vi "Pre Launch Init.vi"(11 "NI_DAQmx(Angular) in":refnum<class "NI_DAQmx(Angular).lvclass">) -> (0 "error out":errorcluster, 3 "NI_DAQmx(Angular) out":refnum<class "NI_DAQmx(Angular).lvclass">)   [LabVIEW 2025, in "NI_DAQmx(Angular).lvclass"]
doc: "<p>(<strong>Filename</strong>: <span class=\"dnl\">Actor Framework.lvlib:Actor.lvclass:Pre Launch Init.vi</span>)</p>\n<p>Defines behavior that occurs after the <a href=\"nihelplauncher://docs/csh?context=lvcore_lvcomm_af_launch_nested_actor\">Launch Nested Actor</a> method is invoked but before the actor's Actor Core method begins running.</p>\n<p>By default, this method does nothing. A descendant class may override it to define behavior.</p>"
uses:
  NI_DAQmx(Angular).lvclass
  NI_DAQmx(Angular).lvclass/NI_DAQmx(Angular).ctl
  DAQ_Abstr/Task_Type/Angular_Task/Angular_Task/Angular_Task.lvclass
  <resource>/objmgr/daqmx.rc
  <vilib>/DAQmx/configure/timing.llb/DAQmx Timing (Sample Clock).vi
  <vilib>/DAQmx/create/channels.llb/DAQmx Create Channel (CI-Position-Angular Encoder).vi
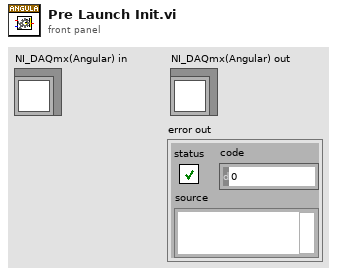
[diagram p1: front panel]
types:
  T1 = typedef "DAQ_Module.lvlib/DAQ_Module.lvclass/DAQ_Task_Config.ctl" = cluster{"Drive":T2, "TaskType":T3, "PhysicalChannels":string, "SampleRateConfiguration":T4, "ChannelConfig":string, "Enable":bool, "ShowPanel":bool}
  T2 = typedef "DAQ_Module.lvlib/DAQ_Module.lvclass/DAQ_HW_Type.ctl" = enum16{"NI_DAQmx", "Simulated_DAQ"}
  T3 = typedef "DAQ_Module.lvlib/DAQ_Module.lvclass/DAQ_Task_Type.ctl" = enum16{"AI", "Linear", "Angular", "AO"}
  T4 = typedef "DAQ_Module.lvlib/DAQ_Module.lvclass/DAQ_SampleRateConfig.ctl" = cluster{"SampleRate":dbl, "SamplesPerChannel":u32, "SamplesPerRead":i32, "SampleMode":i32, "Clock Source":string}
  T5 = typedef "DAQ_Module.lvlib/DAQ_Module.lvclass/DAQ_Angular_Task_Config.ctl" = cluster{"decoding type":i32, "units":i32, "pulses per revolution":u32, "initial angle":dbl, "z index enable":bool, "z index value":dbl, "z index phase":i32, "CI_Encoder_A_InputTerm":string, "CI_Encoder_B_InputTerm":string, "CI_Encoder_Z_InputTerm":string}
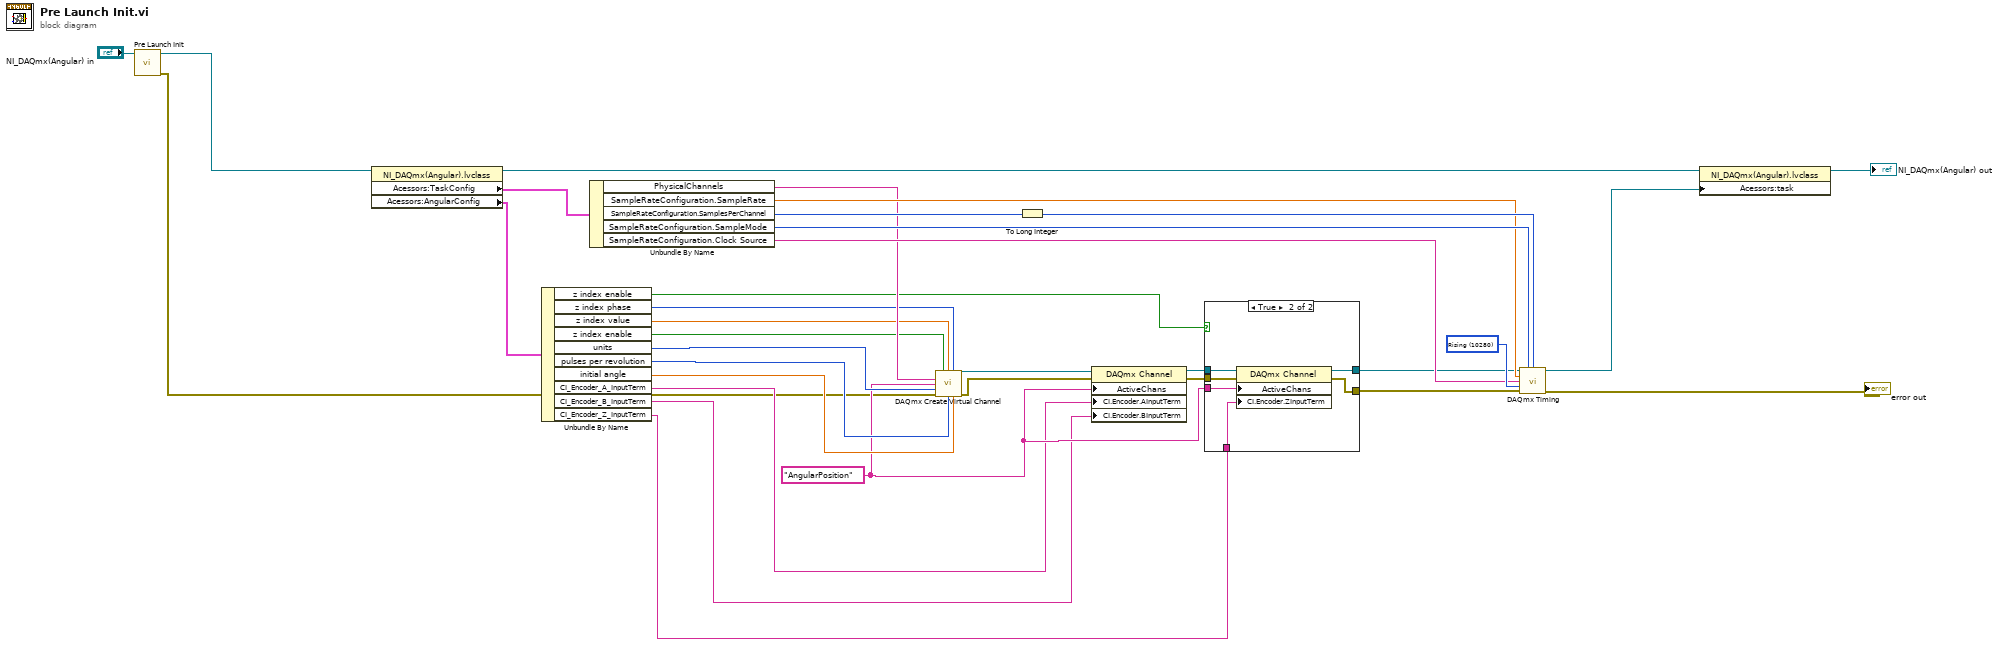
[diagram p0: block diagram]
diagram:
  w8 = "AngularPosition" ("channel name")
  w25 = 10280 items=["Rising"=10280, "Falling"=10171] ("active edge")
  n1 = call-parent "Pre Launch Init.vi"("Task_Abstr in"="NI_DAQmx(Angular) in") -> ("error out"=w1:errorcluster, "Task_Abstr out"=w4:refnum<class "NI_DAQmx(Angular).lvclass">)  [unwired: 9 in]
  n2 = property class="NI_DAQmx(Angular).lvclass"(reference=w4) -> (reference out=w32:refnum<class "NI_DAQmx(Angular).lvclass">, "Acessors:TaskConfig"=w30:T1, "Acessors:AngularConfig"=w31:T5)  [unwired: 1 in, 1 out]
  n3 = Unbundle By Name(w31) -> ("z index enable"=w9:bool, "z index phase"=w21:i32, "z index value"=w20:dbl, "z index enable"=w19:bool, "units"=w18:i32, "pulses per revolution"=w17:u32, "initial angle"=w16:dbl, "CI_Encoder_A_InputTerm"=w7:string, "CI_Encoder_B_InputTerm"=w6:string, "CI_Encoder_Z_InputTerm"=w5:string)
  n4 = Unbundle By Name(w30) -> ("PhysicalChannels"=w22:string, "SampleRateConfiguration.SampleRate"=w26:dbl, "SampleRateConfiguration.SamplesPerChannel"=w28:u32, "SampleRateConfiguration.SampleMode"=w29:i32, "SampleRateConfiguration.Clock Source"=w24:string)
  n5 = call-poly <vilib>:"DAQmx Create Virtual Channel.vi"("z index enable"=w19, "z index value"=w20, "z index phase"=w21, "counter"=w22, "name to assign"=w8, "units"=w18, "error in"=w1, "pulses per revolution"=w17, "initial angle"=w16) -> ("task out"=w13:refnum<k21>, "error out"=w11:errorcluster)  [unwired: 5 in]
  n6 = To Long Integer(number=w28) -> (32bit integer=w27:i32)
  n7 = property class="DAQmx Channel"(reference=w13, error in=w11, "ActiveChans"=w8, "CI.Encoder.AInputTerm"=w7, "CI.Encoder.BInputTerm"=w6) -> (reference out=w15:refnum<k21>, error out=w14:errorcluster)
  n8 = case shown="True" w9 {
    tunnel: w15 -> [w35 w41]
    tunnel: w14 -> [w34 w40]
    tunnel: [w34 w39] -> w10
    tunnel: [w35 w38] -> w12
    tunnel: w8 -> [_ w37]
    tunnel: w5 -> [_ w36]
    frame False {
    }
    frame True {
      n9 = property class="DAQmx Channel"(reference=w41, error in=w40, "ActiveChans"=w37, "CI.Encoder.ZInputTerm"=w36) -> (reference out=w38:refnum<k21>, error out=w39:errorcluster)
    }
  }
  n10 = call-poly <vilib>:"DAQmx Timing.vi"("task/channels in"=w12, "sample mode"=w29, "samples per channel"=w27, "rate"=w26, "source"=w24, "active edge"=w25, "error in"=w10) -> ("task out"=w23:refnum<k21>, "error out"=→"error out":errorcluster)  [unwired: 7 in]
  n11 = property class="NI_DAQmx(Angular).lvclass"(reference=w32, "Acessors:task"=w23) -> (reference out=→"NI_DAQmx(Angular) out":refnum<class "NI_DAQmx(Angular).lvclass">)  [unwired: 1 in, 1 out]
